vi "SParam Limit Testing.vi"(0 "Item Name":string="SDD21", 1 "Frequency":dbl[](array[numeric]), 2 "Pair Name":string="TX1", 3 "specData":string[][](array[string]), 5 "Data In":dbl[](array[numeric])) -> (10 "Next index adder":dbl, 14 "test passed?":bool, 15 "Test Summary":string="SDD21_TX0:OK\rSDD21_TX1:OK\rSDD21_TX2:OK\rSDD21_TX3:OK\rSDD21_RX0:OK\rSDD21_RX1:OK\rSDD21_RX2:OK\rSDD21_RX3:OK\rSDD21 Total Test Result:PASS", 18 "Limit Data":cluster{"Frequency":dbl[], "Data In":dbl[]}[](array[cluster]))   [LabVIEW 2011]
uses:
  <vilib>/measure/mamon.llb/Limit Testing Time.vi
  <vilib>/measure/NI_MAPro.lvlib
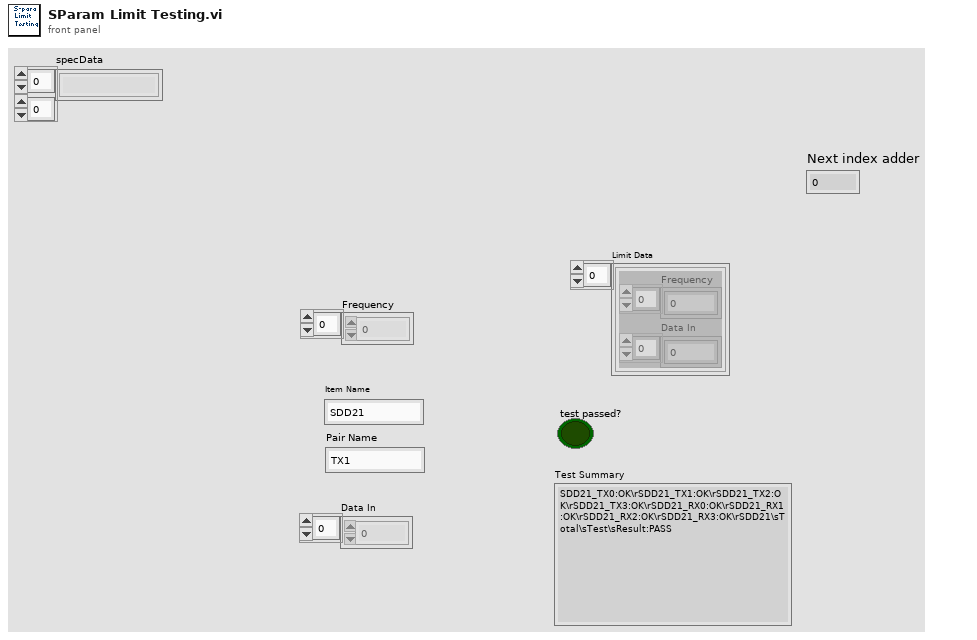
[diagram p1: front panel]
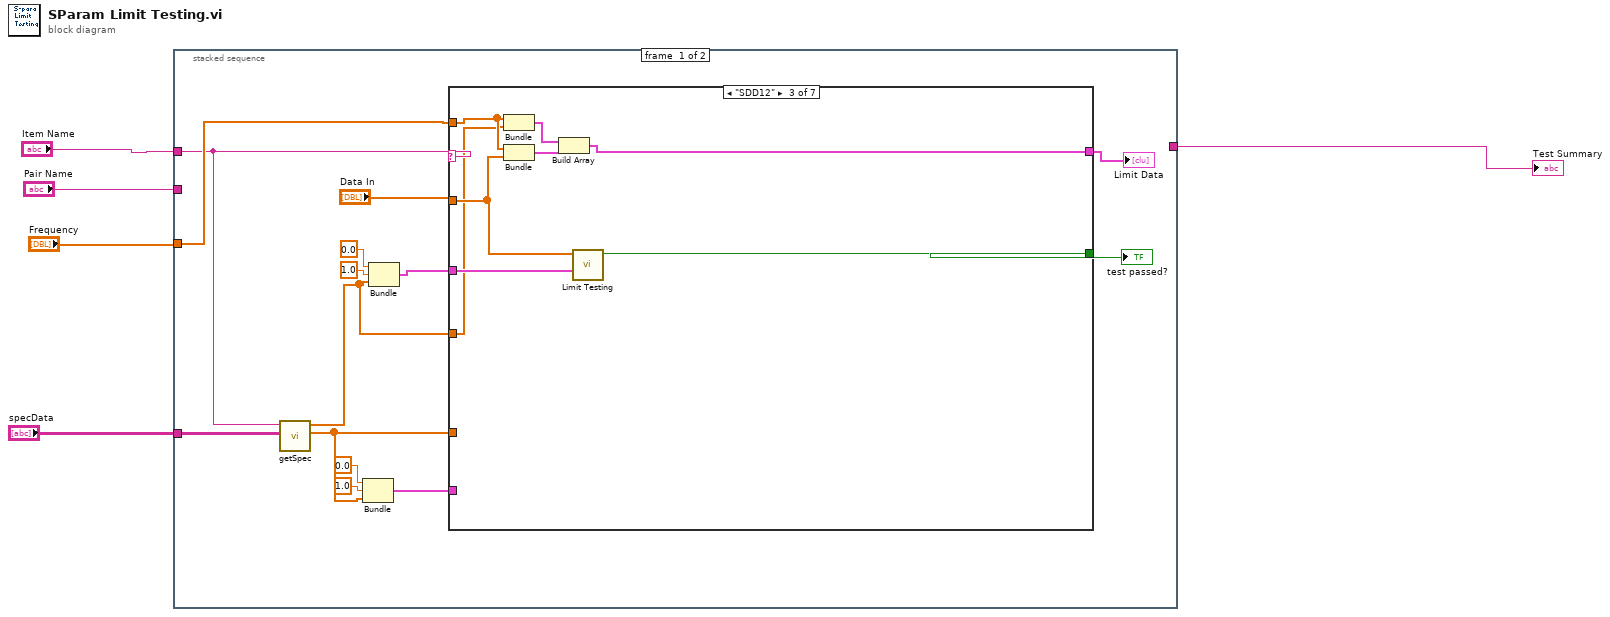
[diagram p0: block diagram]
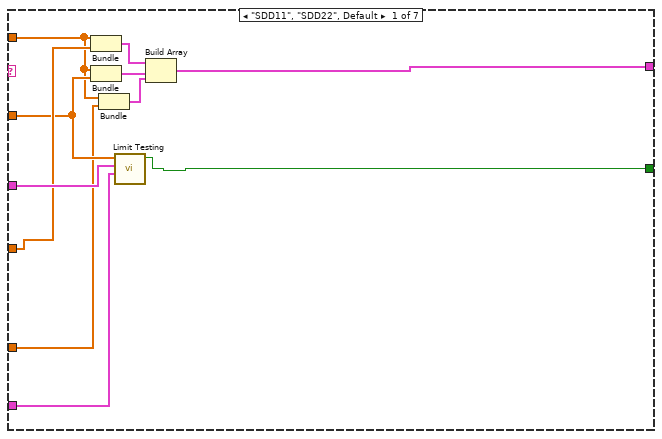
[diagram p2: hidden frame]
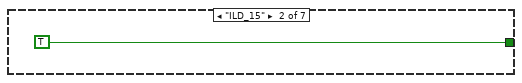
[diagram p3: hidden frame]
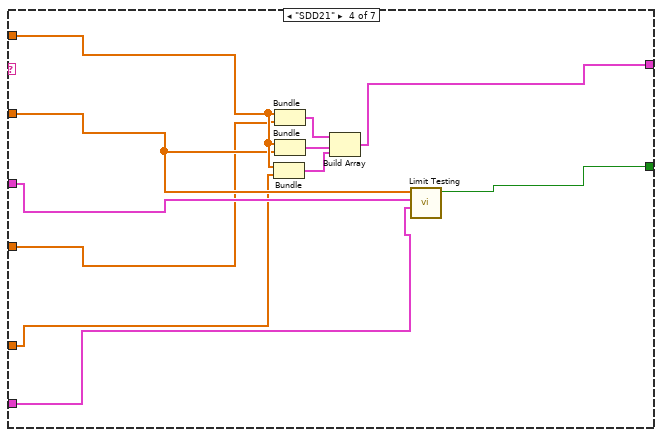
[diagram p4: hidden frame]
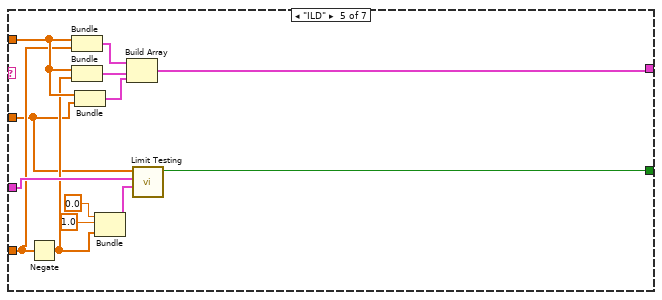
[diagram p5: hidden frame]
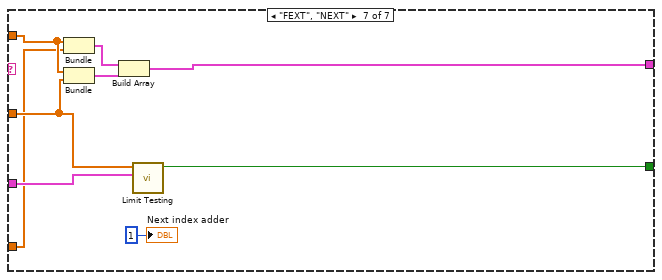
[diagram p7: hidden frame]
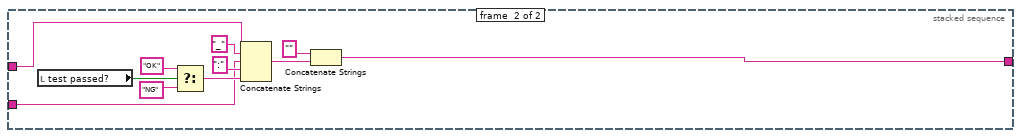
[diagram p8: hidden frame]
diagram:
  n1 = stacked-sequence {
    tunnel: "Item Name" -> [w11 w80]
    tunnel: [_ w74] -> w1
    tunnel: "Pair Name" -> [_ w73]
    tunnel: "Frequency" -> [w14 _]
    tunnel: "specData" -> [w12 _]
    frame #0 {
      n2 = call "getSpec.vi"("specData"=w12, "itemName"=w11) -> ("lowerLimit"=w7:dbl[], "upperLimit"=w10:dbl[])  [unwired: 8 in]
      n3 = Bundle("x0"=0.0, "dx"=1.0, "lowerLimit"=w7) -> (w6:cluster{"x0":dbl, "dx":dbl, "lowerLimit":dbl[]})  [unwired: 1 in]
      n4 = Bundle("x0"=0.0, "dx"=1.0, "upperLimit"=w10) -> (w17:cluster{"x0":dbl, "dx":dbl, "upperLimit":dbl[]})  [unwired: 1 in]
      n5 = case shown="\"SDD12\"" w11 {
        tunnel: w17 -> [w30 _ w38 w49 w62 _ w71]
        tunnel: [w24 TRUE ("test passed?") w39 w50 w63 _ w72] -> w16
        tunnel: "Data In" -> [w26 _ w34 w47 w52 _ w67]
        tunnel: w10 -> [w27 _ w33 w46 w54 _ w66]
        tunnel: w14 -> [w23 _ w35 w48 w56 _ w68]
        tunnel: [w25 _ w32 w45 w51 _ w65] -> w13
        tunnel: w7 -> [w21 _ _ w43 _ _ _]
        tunnel: w6 -> [w20 _ _ w44 _ _ _]
        frame "SDD11", "SDD22", Default {
          n6 = Bundle("Frequency"=w23, "upperLimit"=w27) -> (w28:cluster{"Frequency":dbl[], "upperLimit":dbl[]})  [unwired: 1 in]
          n7 = Bundle("Frequency"=w23, "Data In"=w26) -> (w29:cluster{"Frequency":dbl[], "Data In":dbl[]})  [unwired: 1 in]
          n8 = Bundle("Frequency"=w23, "lowerLimit"=w21) -> (w22:cluster{"Frequency":dbl[], "lowerLimit":dbl[]})  [unwired: 1 in]
          n9 = call-poly <vilib>:"Limit Testing.vi"("lower limit"=w20, "upper limit"=w30, "signal in"=w26) -> ("test passed?"=w24:bool)  [unwired: 3 in, 5 out]
          n10 = Build Array(w28, w29, w22) -> (w25:cluster{"Frequency":dbl[], "lowerLimit":dbl[]}[])
        }
        frame "ILD_15" {
        }
        frame "SDD12" {
          n11 = Bundle("Frequency"=w35, "upperLimit"=w33) -> (w36:cluster{"Frequency":dbl[], "upperLimit":dbl[]})  [unwired: 1 in]
          n12 = Bundle("Frequency"=w35, "Data In"=w34) -> (w37:cluster{"Frequency":dbl[], "Data In":dbl[]})  [unwired: 1 in]
          n13 = Build Array(w36, w37) -> (w32:cluster{"Frequency":dbl[], "Data In":dbl[]}[])
          n14 = call-poly <vilib>:"Limit Testing.vi"("lower limit"=w38, "signal in"=w34) -> ("test passed?"=w39:bool)  [unwired: 4 in, 5 out]
        }
        frame "SDD21" {
          n15 = Bundle("Frequency"=w48, "lowerLimit"=w43) -> (w40:cluster{"Frequency":dbl[], "lowerLimit":dbl[]})  [unwired: 1 in]
          n16 = Bundle("Frequency"=w48, "upperLimit"=w46) -> (w41:cluster{"Frequency":dbl[], "upperLimit":dbl[]})  [unwired: 1 in]
          n17 = Bundle("Frequency"=w48, "Data In"=w47) -> (w42:cluster{"Frequency":dbl[], "Data In":dbl[]})  [unwired: 1 in]
          n18 = Build Array(w41, w42, w40) -> (w45:cluster{"Frequency":dbl[], "lowerLimit":dbl[]}[])
          n19 = call-poly <vilib>:"Limit Testing.vi"("lower limit"=w44, "upper limit"=w49, "signal in"=w47) -> ("test passed?"=w50:bool)  [unwired: 3 in, 5 out]
        }
        frame "ILD" {
          n20 = Negate(x=w54) -> (-x=w53:dbl[])
          n21 = Bundle("Frequency"=w56, "upperLimit"=w54) -> (w57:cluster{"Frequency":dbl[], "upperLimit":dbl[]})  [unwired: 1 in]
          n22 = Bundle("Frequency"=w56, w53) -> (w58:cluster{"Frequency":dbl[], dbl[]})  [unwired: 1 in]
          n23 = Bundle("Frequency"=w56, "Data In"=w52) -> (w55:cluster{"Frequency":dbl[], "Data In":dbl[]})  [unwired: 1 in]
          n24 = Bundle("x0"=0.0, "dx"=1.0, w53) -> (w59:cluster{"x0":dbl, "dx":dbl, dbl[]})  [unwired: 1 in]
          n25 = Build Array(w57, w58, w55) -> (w51:cluster{"Frequency":dbl[], "Data In":dbl[]}[])
          n26 = call-poly <vilib>:"Limit Testing.vi"("lower limit"=w59, "upper limit"=w62, "signal in"=w52) -> ("test passed?"=w63:bool)  [unwired: 3 in, 5 out]
        }
        frame "TDD11", "TDD22" {
        }
        frame "FEXT", "NEXT" {
          n27 = Bundle("Frequency"=w68, "upperLimit"=w66) -> (w69:cluster{"Frequency":dbl[], "upperLimit":dbl[]})  [unwired: 1 in]
          n28 = Bundle("Frequency"=w68, "Data In"=w67) -> (w70:cluster{"Frequency":dbl[], "Data In":dbl[]})  [unwired: 1 in]
          n29 = Build Array(w69, w70) -> (w65:cluster{"Frequency":dbl[], "Data In":dbl[]}[])
          n30 = call-poly <vilib>:"Limit Testing.vi"("upper limit"=w71, "signal in"=w67) -> ("test passed?"=w72:bool)  [unwired: 4 in, 5 out]
          "Next index adder" <- 1
        }
      }
      "test passed?" <- w16
      "Limit Data" <- w13
    }
    frame #1 {
      n31 = local read "test passed?"() -> (w75:bool)
      n32 = Select(t="OK", s=w75, f="NG") -> (s? t:f=w77:string)
      n33 = Concatenate Strings(w80, "_" ("字符串"), w73, ":" ("字符串"), w77) -> (w76:string)
      n34 = Concatenate Strings("", w76) -> (w74:string)
    }
  }
  "Test Summary" <- w1
